vi "Step.GetProperties.vi"(11 "String in":string) -> (1 "Warning":string, 2 "Parameters":dbl[](array[numeric]), 3 "Step":T1)   [LabVIEW 2013, in "Simple Sequence Tools - Shared.lvlib"]
uses:
  Simple Sequence Tools - Shared.lvlib
  Types/StepTypes.ctl
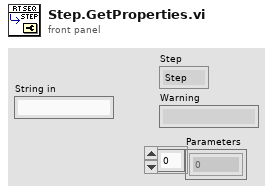
[diagram p1: front panel]
types:
  T1 = typedef "Simple Sequence Tools - Shared.lvlib/StepTypes.ctl" = enum8{"Step", "iStep", "Ramp", "Unchanged", "Unknown"}
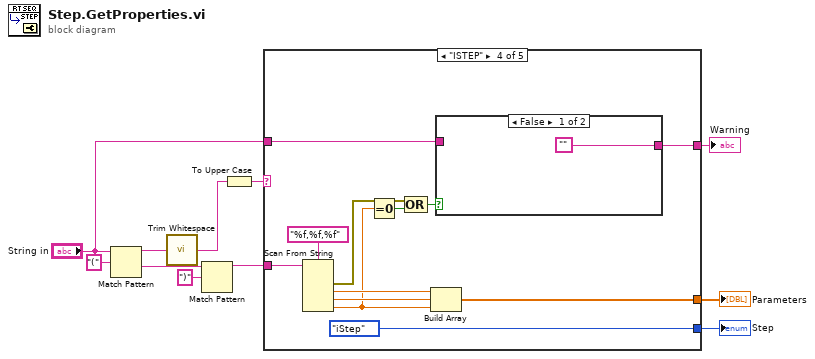
[diagram p0: block diagram]
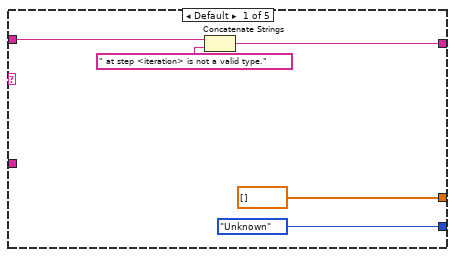
[diagram p2: hidden frame]
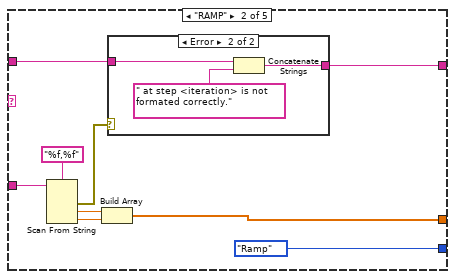
[diagram p3: hidden frame]
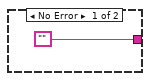
[diagram p4: hidden frame]
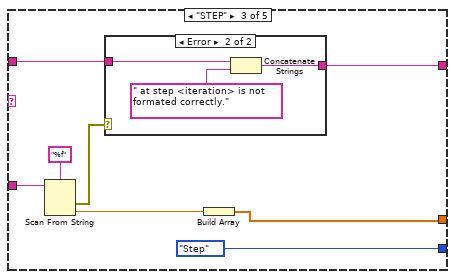
[diagram p5: hidden frame]
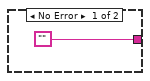
[diagram p6: hidden frame]
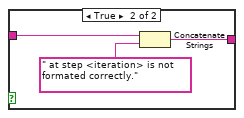
[diagram p7: hidden frame]
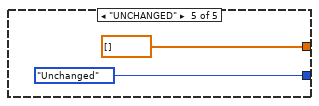
[diagram p8: hidden frame]
diagram:
  n1 = Match Pattern(string="String in", regular expression="(") -> (before substring=w8:string, after substring=w9:string)  [unwired: 1 in, 2 out]
  n2 = call <vilib>:"Trim Whitespace.vi"("string"=w8) -> ("trimmed string"=w11:string)  [unwired: 1 in]
  n3 = Match Pattern(string=w9, regular expression=")") -> (before substring=w4:string)  [unwired: 1 in, 3 out]
  n4 = To Upper Case(1:w11) -> (0:w6:string)
  n5 = case shown="\"ISTEP\"" w6 {
    tunnel: [StepTypes."Unknown" StepTypes."Ramp" StepTypes."Step" StepTypes."iStep" StepTypes."Unchanged"] -> w5
    tunnel: w4 -> [_ w22 w36 w50 _]
    tunnel: [dbl[] [] w20 w33 w48 dbl[] []] -> w3
    tunnel: "String in" -> [w14 w18 w31 w46 _]
    tunnel: [w12 w17 w30 w45 _] -> w1
    frame Default {
      n6 = Concatenate Strings(w14, " at step <iteration> is not a valid type.") -> (w12:string)
    }
    frame "RAMP" {
      n7 = Scan From String(format string="%f,%f", input string=w22) -> (error out=w19:errorcluster, output 1=w23:dbl, output 2=w21:dbl)  [unwired: 4 in, 2 out]
      n8 = Build Array(w23, w21) -> (w20:dbl[])
      n9 = case shown="Error" w19 {
        tunnel: w18 -> [_ w28]
        tunnel: ["" w27] -> w17
        frame No Error {
        }
        frame Error {
          n10 = Concatenate Strings(w28, " at step <iteration> is not formated correctly.") -> (w27:string)
        }
      }
    }
    frame "STEP" {
      n11 = Scan From String(format string="%f", input string=w36) -> (error out=w32:errorcluster, output 1=w34:dbl)  [unwired: 3 in, 2 out]
      n12 = case shown="Error" w32 {
        tunnel: w31 -> [_ w40]
        tunnel: ["" w39] -> w30
        frame No Error {
        }
        frame Error {
          n13 = Concatenate Strings(w40, " at step <iteration> is not formated correctly.") -> (w39:string)
        }
      }
      n14 = Build Array(w34) -> (w33:dbl[])
    }
    frame "ISTEP" {
      n15 = Scan From String(format string="%f,%f,%f", input string=w50) -> (error out=w47:errorcluster, output 1=w51:dbl, output 2=w49:dbl, output 3=w43:dbl)  [unwired: 5 in, 2 out]
      n16 = Equal To 0?(x=w43) -> (x = 0?=w42:bool)
      n17 = Compound Arithmetic op=OR(w47, w42) -> (w44:bool)
      n18 = Build Array(w51, w49, w43) -> (w48:dbl[])
      n19 = case shown="False" w44 {
        tunnel: w46 -> [_ w56]
        tunnel: ["" w55] -> w45
        frame False {
        }
        frame True {
          n20 = Concatenate Strings(w56, " at step <iteration> is not formated correctly.") -> (w55:string)
        }
      }
    }
    frame "UNCHANGED" {
    }
  }
  "Parameters" <- w3
  "Step" <- w5
  "Warning" <- w1
